vi "报警时间设置读取与保存 (子VI).vi"(8 "值in":bool, 9 "有in":T1, 10 "无in":T1, 11 "枚举":enum16{"读取", "写入屏蔽蜂鸣器", "写入报警时间设置"}(ring)) -> (1 "值out":bool, 2 "有out":T1, 3 "无out":T1)   [LabVIEW 2017]
uses:
  <vilib>/Utility/file.llb/Write Delimited Spreadsheet (DBL).vi
  <vilib>/Utility/file.llb/Read Delimited Spreadsheet (DBL).vi
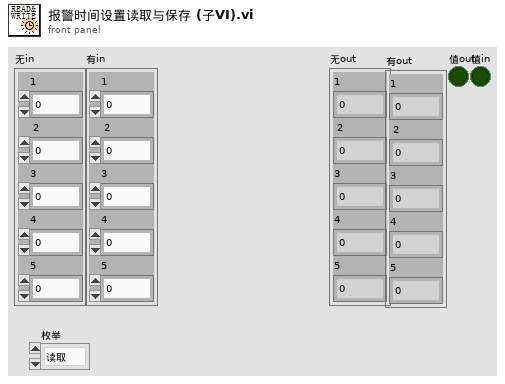
[diagram p1: front panel]
types:
  T1 = cluster{"1":dbl, " 2":dbl, "3":dbl, "4":dbl, "5":dbl}
  T2 = cluster{"all rows[0]":dbl, "all rows[1]":dbl, "all rows[2]":dbl, "all rows[3]":dbl, "all rows[4]":dbl}
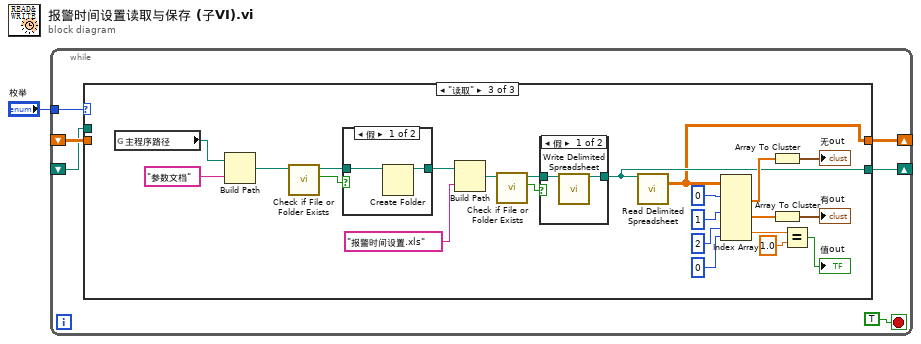
[diagram p0: block diagram]
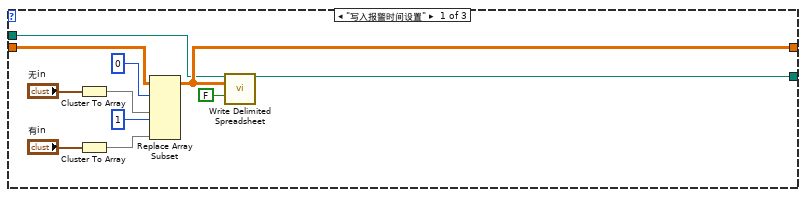
[diagram p2: hidden frame]
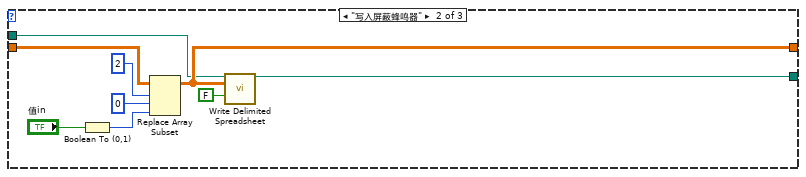
[diagram p3: hidden frame]
diagram:
  n1 = while {
    tunnel: "枚举" -> [w7]
    shift-right: [w6] -> _
    shift-left: _ -> [w2]
    shift-right: [w5] -> _
    shift-left: _ -> [w3]
    stop <- TRUE stop-if-true
    n2 = case shown="\"读取\"" w7 {
      tunnel: [w12 w24 w32] -> w6
      tunnel: [w13 w23 w31] -> w5
      tunnel: w3 -> [w18 w27 _]
      tunnel: w2 -> [w11 w21 _]
      frame "写入报警时间设置" {
        n3 = Cluster To Array(cluster="无in") -> (array=w16:dbl[])
        n4 = Cluster To Array(cluster="有in") -> (array=w14:dbl[])
        n5 = Replace Array Subset(array=w18, new element #1=w16, index (row) #1=0 ("索引 (行)"), new element #2=w14, index (row) #2=1 ("索引 (行)")) -> (w13:dbl[][])  [unwired: 2 in]
        n6 = call-poly <vilib>:"Write Delimited Spreadsheet.vi"("file path (dialog if empty)"=w11, "2D data"=w13, "append to file? (new file:F)"=FALSE) -> ("new file path (Not A Path if cancelled)"=w12:path)  [unwired: 11 in, 1 out]
      }
      frame "写入屏蔽蜂鸣器" {
        n7 = Boolean To (0,1)(Boolean="值in") -> (0, 1=w22:i16)
        n8 = Replace Array Subset(array=w27, new element=w22, index (row)=2 ("索引 (行)"), index (col)=0 ("禁用的索引 (列)")) -> (w23:dbl[][])
        n9 = call-poly <vilib>:"Write Delimited Spreadsheet.vi"("file path (dialog if empty)"=w21, "2D data"=w23, "append to file? (new file:F)"=FALSE) -> ("new file path (Not A Path if cancelled)"=w24:path)  [unwired: 11 in, 1 out]
      }
      frame "读取" {
        n10 = global read "全局 1.vi" "主程序路径"() -> (w50:path)
        n11 = Build Path(base path=w50, name or relative path="参数文档" ("名称或相对路径")) -> (appended path=w47:path)
        n12 = call <vilib>:"Check if File or Folder Exists.vi"("path"=w47) -> ("file or folder exists?"=w48:bool, "dup path"=w46:path)  [unwired: 8 in, 1 out]
        n13 = case shown="假" w48 {
          tunnel: w46 -> [w55 w56]
          tunnel: [w54 w56] -> w45
          frame False {
            n14 = Create Folder(path (use dialog)=w55) -> (created path=w54:path)  [unwired: 2 in, 2 out]
          }
          frame True {
          }
        }
        n15 = Build Path(base path=w45, name or relative path="报警时间设置.xls" ("名称或相对路径")) -> (appended path=w43:path)
        n16 = call <vilib>:"Check if File or Folder Exists.vi"("path"=w43) -> ("file or folder exists?"=w42:bool, "dup path"=w41:path)  [unwired: 8 in, 1 out]
        n17 = case shown="假" w42 {
          tunnel: w41 -> [w52 w53]
          tunnel: [w51 w53] -> w32
          frame False {
            n18 = call-poly <vilib>:"Write Delimited Spreadsheet.vi"("file path (dialog if empty)"=w52) -> ("new file path (Not A Path if cancelled)"=w51:path)  [unwired: 13 in, 1 out]
          }
          frame True {
          }
        }
        n19 = call-poly <vilib>:"Read Delimited Spreadsheet.vi"("file path (dialog if empty)"=w32) -> ("all rows"=w31:dbl[][])  [unwired: 9 in, 5 out]
        n20 = Index Array(array=w31, index (row) #1=0 ("索引 (行)"), index (row) #2=1 ("索引 (行)"), index (row) #3=2 ("索引 (行)"), index (col) #3=0 ("禁用的索引 (列)")) -> (element #1=w37:dbl[], element #2=w36:dbl[], element #3=w34:dbl)  [unwired: 2 in]
        n21 = Array To Cluster(array=w37) -> (cluster=→"无out":T2)
        n22 = Array To Cluster(array=w36) -> (cluster=→"有out":T2)
        n23 = Equal?(x=w34, y=1.0) -> (x = y?=→"值out":bool)
      }
    }
  }
